vi "Compile Battery Switch.vi"(8 "error in (no error)":errorcluster, 10 "Name":string, 11 "Device Item Ref in":T5 format="%.0x") -> (0 "error out":errorcluster, 1 "Battery Switch Engine Data":T1 {"Ordered Channels" format="%.0x"; "RT IDs"."Slot #" max=15; "RT IDs"."Chip Address (A2 A1 A0)" max=7}, 2 "Initial Battery Switch SPI CMDs":u64[](array[numeric]), 3 "Device Item Ref out":T5 format="%.0x")   [LabVIEW 2014, in "SLSC configuration Shared.lvlib"]
uses:
  Shared/SLSC configuration Shared.lvlib
  <vilib>/NI Veristand/Custom Device API/Custom Device Item Ref.ctl
  Shared/Type Defs/RT Engine Data.ctl
  Shared/Type Defs/RT IDs.ctl
  Shared/SPI Utility/Slot #.ctl
  Shared/MCP23S17/Chip Address.ctl
  Shared/Constants.vi
  <vilib>/NI Veristand/Custom Device Tools/Custom Device Utility Library/Custom Device Utility Library.lvlib
  <vilib>/NI Veristand/Custom Device API/Custom Device API.lvlib
  SLSC configuration System Explorer.lvlib
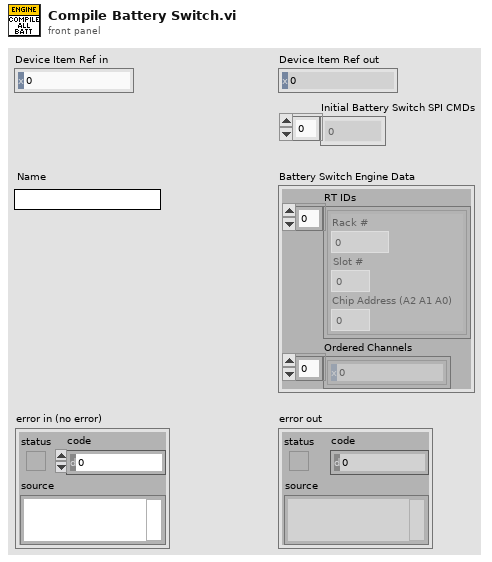
[diagram p1: front panel]
types:
  T1 = typedef "SLSC configuration Shared.lvlib/RT Engine Data.ctl" = cluster{"RT IDs":T2[], "Ordered Channels":T5[]}
  T2 = typedef "SLSC configuration Shared.lvlib/RT IDs.ctl" = cluster{"Rack #":u8, "Slot #":T3, "Chip Address (A2 A1 A0)":T4}
  T3 = typedef "SLSC configuration Shared.lvlib/Slot #.ctl" = u8
  T4 = typedef "SLSC configuration Shared.lvlib/Chip Address.ctl" = u8
  T5 = typedef "Custom Device API.lvlib/Custom Device Item Ref.ctl" = u64
  T6 = typedef "SLSC configuration Shared.lvlib/Card Position.ctl" = cluster{"Rack #":u8, "Slot #":T3}
  T7 = typedef "SLSC configuration Shared.lvlib/Battery Switch.ctl" = enum8{"Off", "On"}
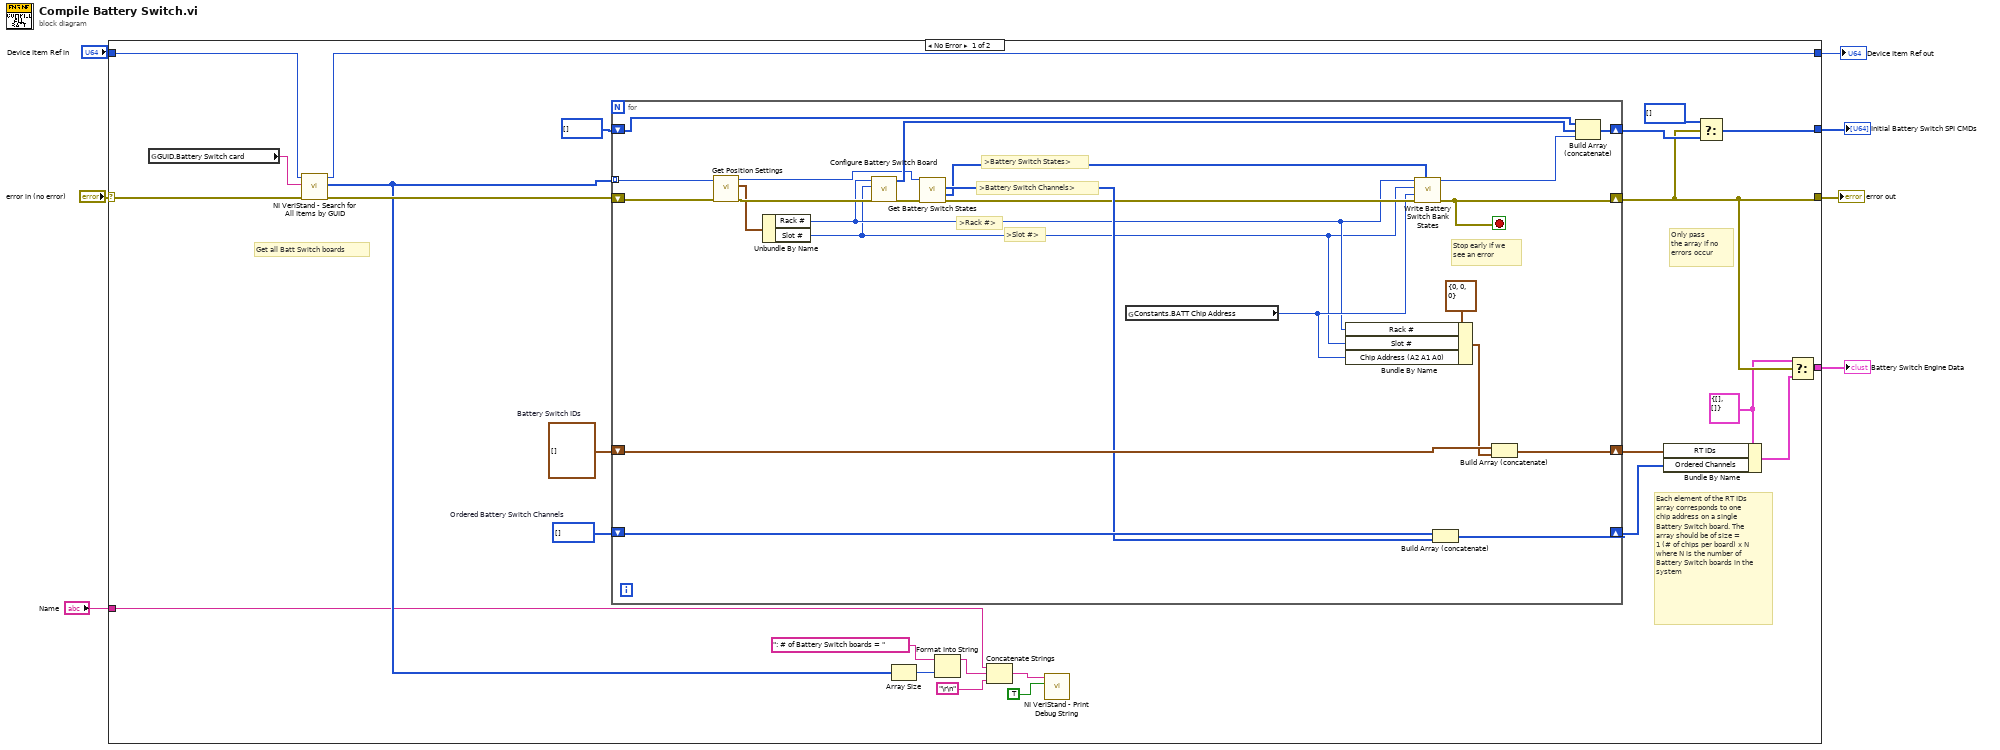
[diagram p0: block diagram]
diagram:
  n1 = case shown="No Error" "error in (no error)" {
    selector: "error in (no error)" -> [w30 w57]
    tunnel: [w19 w57] -> w7
    tunnel: "Device Item Ref in" -> [w24 w56]
    tunnel: [w16 _] -> w4
    tunnel: [w20 _] -> w3
    tunnel: [w23 w56] -> w2
    tunnel: "Name" -> [w8 _]
    frame No Error {
      w18 = T1 {"RT IDs"=[], "Ordered Channels"=[]} ("FIU Engine Data")
      w27 = T5[] []  # Ordered Battery Switch Channels
      w28 = T2[] []  # Battery Switch IDs
      # "Only pass\nthe array if no\nerrors occur"
      # "Get all Batt Switch boards"
      # "Each element of the RT IDs array corresponds to one chip address on a single Battery Switch board. The array should be of size =\n1 (# of chips per board) x N where N is the number of Battery Switch boards in the system"
      n2 = global read "Constants.vi" "GUID.Battery Switch card"() -> (w32:string)
      n3 = call <vilib>:"NI VeriStand - Search for All Items by GUID.vi"("error in"=w30, "Item GUID"=w32, "Section Ref in"=w24) -> ("error out"=w31:errorcluster, "Item Refs"=w9:T5[], "Section Ref out"=w23:T5)  [unwired: 5 in, 1 out]
      n4 = for {
        tunnel: w9 -> [w39] mode=indexing
        shift-right: [w44] -> w19
        shift-left: w31 -> [w38]
        shift-right: [w51] -> w22
        shift-left: u64[] [] ("SPI FIFO Messages") -> [w55]
        shift-right: [w49] -> w26
        shift-left: w28 -> [w50]
        shift-right: [w47] -> w25
        shift-left: w27 -> [w48]
        stop <- w44 stop-if-true
        # ">Battery Switch States>"
        # "Stop early if we\nsee an error"
        # ">Battery Switch Channels>"
        # ">Slot #>"
        # ">Rack #>"
        n5 = call "Get Position Settings.vi"("error in (no error)"=w38, "Item Ref in"=w39) -> ("error out"=w37:errorcluster, "Card Position"=w35:T6, "Item Ref out"=w36:T5)  [unwired: 7 in]
        n6 = Unbundle By Name(w35) -> ("Rack #"=w34:u8, "Slot #"=w33:T3)
        n7 = call "Configure Battery Switch Board.vi"("error in (no error)"=w37, "Slot #"=w33, "Rack #"=w34) -> ("error out"=w53:errorcluster, "SPI FIFO Messages"=w54:u64[])  [unwired: 7 in]
        n8 = call "Get Battery Switch States.vi"("error in (no error)"=w53, "Item Ref in"=w36) -> ("error out"=w45:errorcluster, "Battery Switch States"=w42:T7[], "Ordered Battery Switch Channels"=w46:T5[])  [unwired: 6 in, 1 out]
        n9 = global read "Constants.vi" "Constants.BATT Chip Address"() -> (w43:u8)
        n10 = Bundle By Name(cluster=T2 {"Rack #"=0, "Slot #"=0, "Chip Address (A2 A1 A0)"=0}, "Rack #"=w34, "Slot #"=w33, "Chip Address (A2 A1 A0)"=w43) -> (w40:T2)
        n11 = call "Write Battery Switch Bank States.vi"("Battery Switch States"=w42, "error in (no error)"=w45, "Chip Address (A2 A1 A0)"=w43, "Slot #"=w33, "Rack #"=w34) -> ("error out"=w44:errorcluster, "FIFO SPI Message"=w52:u64)  [unwired: 4 in, 1 out]
        n12 = Build Array (concatenate)(w48, w46) -> (w47:T5[])
        n13 = Build Array (concatenate)(w50, w40) -> (w49:T2[])
        n14 = Build Array (concatenate)(w55, w54, w52) -> (w51:u64[])
      }
      n15 = Array Size(array=w9) -> (size(s)=w14:i32)
      n16 = Format Into String(initial string=": # of Battery Switch boards = ", w14) -> (resulting string=w11:string)  [unwired: 2 in, 1 out]
      n17 = Concatenate Strings(w8, w11, "\r\n") -> (w12:string)
      n18 = call <vilib>:"NI VeriStand - Print Debug String.vi"("Add to log file? (T)"=TRUE, "Message"=w12) -> ()  [unwired: 9 in, 1 out]
      n19 = Bundle By Name(cluster=w18, "RT IDs"=w26, "Ordered Channels"=w25) -> (w17:T1)
      n20 = Select(t=u64[] [], s=w19, f=w22) -> (s? t:f=w20:u64[])
      n21 = Select(t=w18, s=w19, f=w17) -> (s? t:f=w16:T1)
    }
    frame Error {
    }
  }
  "error out" <- w7
  "Device Item Ref out" <- w2
  "Battery Switch Engine Data" <- w4
  "Initial Battery Switch SPI CMDs" <- w3
